vi "Check Fcn and Dev Selection requested by UI.vi"(6 "Master?":bool, 8 "error in (no error)":errorcluster, 9 "DevInfos":refnum<class "DevInfo.lvclass">[](array[class]), 10 "Function Name":string, 11 "Controller in":refnum<class "Controller.lvclass">) -> (0 "error out":errorcluster, 2 "valid":bool, 3 "Controller out":refnum<class "Controller.lvclass">)   [LabVIEW 2016, in "Controller Actor.lvlib" / "Controller.lvclass"]
uses:
  <userlib>/Common Components/Controller/Controller.lvclass
  C:/Program Files (x86)/National Instruments/LabVIEW 2016/vi.lib/ActorFramework/Actor/Actor.lvclass
  <userlib>/Common Components/Hardware/DevInfo/DevInfo.lvclass
  <vilib>/ActorFramework/Actor/Actor.lvclass/Actor.ctl
  <vilib>/ActorFramework/Message Enqueuer/Message Enqueuer.lvclass/Message Enqueuer.ctl
  <vilib>/ActorFramework/Message Enqueuer/Init from Existing Queue.vi
  <vilib>/ActorFramework/Message Enqueuer/Message Enqueuer.lvclass
  <userlib>/Common Components/Controller UI/Messages/Check Run Button/Check Validity of Selection.lvclass
  <vilib>/ActorFramework/Actor/Actor.lvclass
  <userlib>/Common Components/Controller/Messages/Log Status/Log Status.lvclass
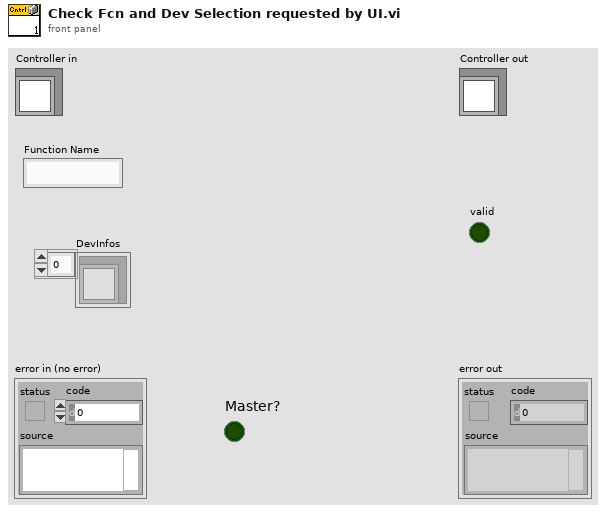
[diagram p1: front panel]
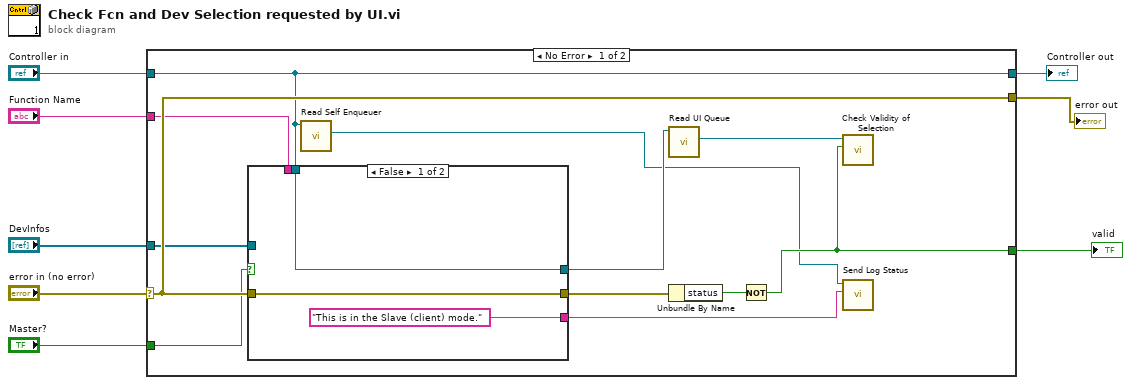
[diagram p0: block diagram]
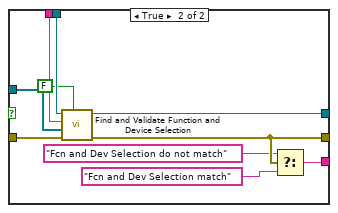
[diagram p2: hidden frame]
diagram:
  n1 = case shown="No Error" "error in (no error)" {
    selector: "error in (no error)" -> [w20 w35]
    tunnel: [w20 w35] -> w7
    tunnel: [w13 w34] -> w5
    tunnel: "Controller in" -> [w13 w34]
    tunnel: "Function Name" -> [w19 _]
    tunnel: "DevInfos" -> [w18 _]
    tunnel: [w12 _] -> w2
    tunnel: "Master?" -> [w10 _]
    frame No Error {
      n2 = case shown="False" w10 {
        tunnel: w20 -> [w22 w33]
        tunnel: w19 -> [_ w32]
        tunnel: w18 -> [_ w31]
        tunnel: [w23 w30] -> w17
        tunnel: [w22 w27] -> w16
        tunnel: w13 -> [w23 w29]
        tunnel: ["This is in the Slave (client) mode." w24] -> w9
        frame False {
        }
        frame True {
          n3 = call <userlib>:"Find and Validate Function and Device Selection.vi"("reserve?"=FALSE, "error in (no error)"=w33, "DevInfos"=w31, "Function Name"=w32, "Controller in"=w29) -> ("error out"=w27:errorcluster, "Controller out"=w30:refnum<class "Controller.lvclass">)  [unwired: 3 in, 2 out]
          n4 = Select(t="Fcn and Dev Selection do not match", s=w27, f="Fcn and Dev Selection match") -> (s? t:f=w24:string)
        }
      }
      n5 = call <vilib>:"Read Self Enqueuer.vi"("Actor"=w13) -> ("Self Enqueuer"=w11:refnum<class "Message Enqueuer.lvclass">)  [unwired: 10 in]
      n6 = call <userlib>:"Read UI Queue.vi"("UI Controller in"=w17) -> ("UI Queue"=w14:refnum<class "Message Enqueuer.lvclass">)  [unwired: 8 in, 2 out]
      n7 = Unbundle By Name(w16) -> ("status"=w15:bool)
      n8 = Not(x=w15) -> (.not. x?=w12:bool)
      n9 = call <userlib>:"Check Validity of Selection.vi"("valid"=w12, "Message Enqueuer in"=w14) -> ()  [unwired: 8 in, 2 out]
      n10 = call <userlib>:"Send Log Status.vi"("String"=w9, "Message Enqueuer in"=w11) -> ()  [unwired: 8 in, 2 out]
    }
    frame Error {
    }
  }
  "error out" <- w7
  "Controller out" <- w5
  "valid" <- w2
